vi "Agilent DMM Set Range.vi"(7 "Measurement Type":T2, 8 "error in (no error)":errorcluster, 10 "Range":T1, 11 "VISA Resource Name":refnum<visa-resource-name>) -> (0 "error out":errorcluster, 3 "dup VISA Resource Name":refnum<visa-resource-name>)   [LabVIEW 2011]
doc: "This VI for the HP 8753 is used to read the sweep type.\n\n0 LINEAR FREQ\n1 LOG FREQ\n2 LIST FREQ\n3 CW TIME\n4 POWER SWEEP"
uses:
  TypeDefs/Agilent DMM Measurement Type.ctl
  TypeDefs/Agilent DMM Range.ctl
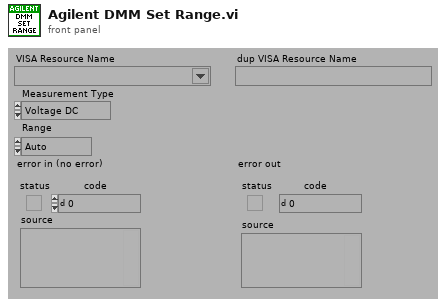
[diagram p1: front panel]
types:
  T1 = typedef "Agilent DMM Range.ctl" = enum16{"Auto", "Min", "Max", "0.01", "0.1", "1", "3", "10", "100", "1,000", "10,000", "100,000", "1,000,000", "10,000,000", "100,000,000"}
  T2 = typedef "Agilent DMM Measurement Type.ctl" = enum16{"Voltage DC", "Voltage DC Ratio", "Voltage AC", "Current DC", "Current AC", "Resistance", "Fresistance", "Frequency", "Period", "Continuity", "Diode"}
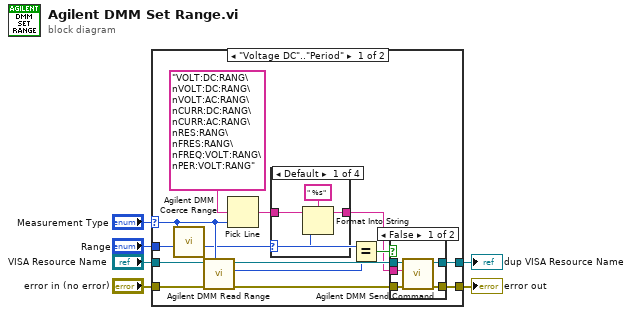
[diagram p0: block diagram]
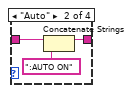
[diagram p3: hidden frame]
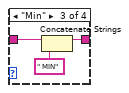
[diagram p4: hidden frame]
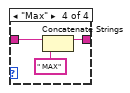
[diagram p5: hidden frame]
diagram:
  n1 = case shown="\"Voltage DC\"..\"Period\"" "Measurement Type" {
    selector: "Measurement Type" -> [w15 _]
    tunnel: "error in (no error)" -> [w17 w42]
    tunnel: [w10 w42] -> w5
    tunnel: "VISA Resource Name" -> [w16 w41]
    tunnel: [w11 w41] -> w3
    tunnel: "Range" -> [w18 _]
    frame "Voltage DC".."Period" {
      n2 = call "Agilent DMM Coerce Range.vi"("Range"=w18, "Measurement Type"=w15) -> ("Coerced Range"=w7:T1)  [unwired: 9 out]
      n3 = call "Agilent DMM Read Range.vi"("Measurement Type"=w15, "error in (no error)"=w17, "VISA Resource Name"=w16) -> ("error out"=w13:errorcluster, "Range"=w9:T1, "dup VISA Resource Name"=w12:refnum<visa-resource-name>)  [unwired: 6 out]
      n4 = Pick Line(multi-line string="VOLT:DC:RANG\nVOLT:DC:RANG\nVOLT:AC:RANG\nCURR:DC:RANG\nCURR:AC:RANG\nRES:RANG\nFRES:RANG\nFREQ:VOLT:RANG\nPER:VOLT:RANG" ("write buffer"), line index=w15) -> (output string=w19:string)  [unwired: 1 out]
      n5 = case shown="Default" w7 {
        selector: w7 -> [w28 _ _ _]
        tunnel: w19 -> [w29 w33 w36 w39]
        tunnel: [w30 w34 w37 w40] -> w8
        frame Default {
          n6 = Format Into String(format string=" %s", initial string=w29, w28) -> (resulting string=w30:string)  [unwired: 1 in, 1 out]
        }
        frame "Auto" {
          n7 = Concatenate Strings(w33, ":AUTO ON" ("format string")) -> (w34:string)
        }
        frame "Min" {
          n8 = Concatenate Strings(w36, " MIN" ("format string")) -> (w37:string)
        }
        frame "Max" {
          n9 = Concatenate Strings(w39, " MAX" ("format string")) -> (w40:string)
        }
      }
      n10 = Equal?(x=w7, y=w9) -> (x = y?=w14:bool)
      n11 = case shown="False" w14 {
        tunnel: [w25 w27] -> w11
        tunnel: [w24 w26] -> w10
        tunnel: w8 -> [w23 _]
        tunnel: w12 -> [w22 w27]
        tunnel: w13 -> [w21 w26]
        frame False {
          n12 = call "Agilent DMM Send Command.vi"("error in (no error)"=w21, "Command"=w23, "VISA Resource Name"=w22) -> ("error out"=w24:errorcluster, "dup VISA Resource Name"=w25:refnum<visa-resource-name>)  [unwired: 2 in, 5 out]
        }
        frame True {
        }
      }
    }
    frame Default {
      # "The Range can not be set for:\n\nContinuity, or Diode."
    }
  }
  "dup VISA Resource Name" <- w3
  "error out" <- w5
